vi "Update Values VI.vi"(4 "Project Ref":refnum<vi>, 6 "Names":string[](array[string]), 7 "Entity Paths":T1, 8 "error in (no error)":errorcluster) -> (0 "error":errorcluster)   [LabVIEW 2020, in "Conditum-Tools.lvlib" / "Entity Editor.lvclass"]
uses:
  Entity Editor.lvclass
  Entity Paths.ctl
  <vilib>/Utility/miscctls.llb/LVPositionTypeDef.ctl
  <vilib>/Utility/traverseref.llb/TRef TravTarget.ctl
  <vilib>/IlluminatedG/IG Conditum Base/Conditum/Columns/Type/Copy Value.vi
  <vilib>/Utility/traverseref.llb/VI Scripting - Traverse.lvlib
  <vilib>/IlluminatedG/IG Conditum Base/Conditum/Columns/Type/Type.lvclass
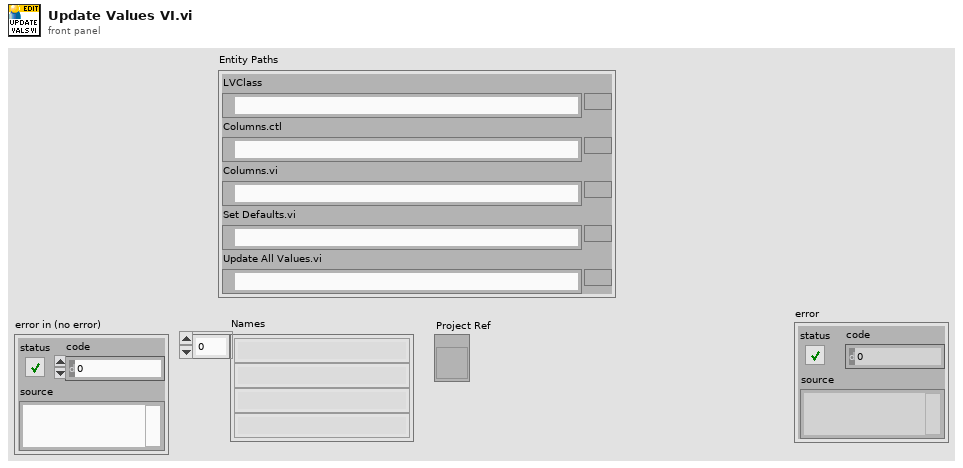
[diagram p1: front panel]
types:
  T1 = typedef "Conditum-Tools.lvlib/Entity Editor.lvclass/Entity Paths.ctl" = cluster{"LVClass":path, "Columns.ctl":path, "Columns.vi":path, "Set Defaults.vi":path, "Update All Values.vi":path}
  T2 = typedef "TRef TravTarget.ctl" = enum16{"FP", "BD", "Other"}
  T3 = typedef "LVPositionTypeDef.ctl" = cluster{"Left":i32, "Top":i32}
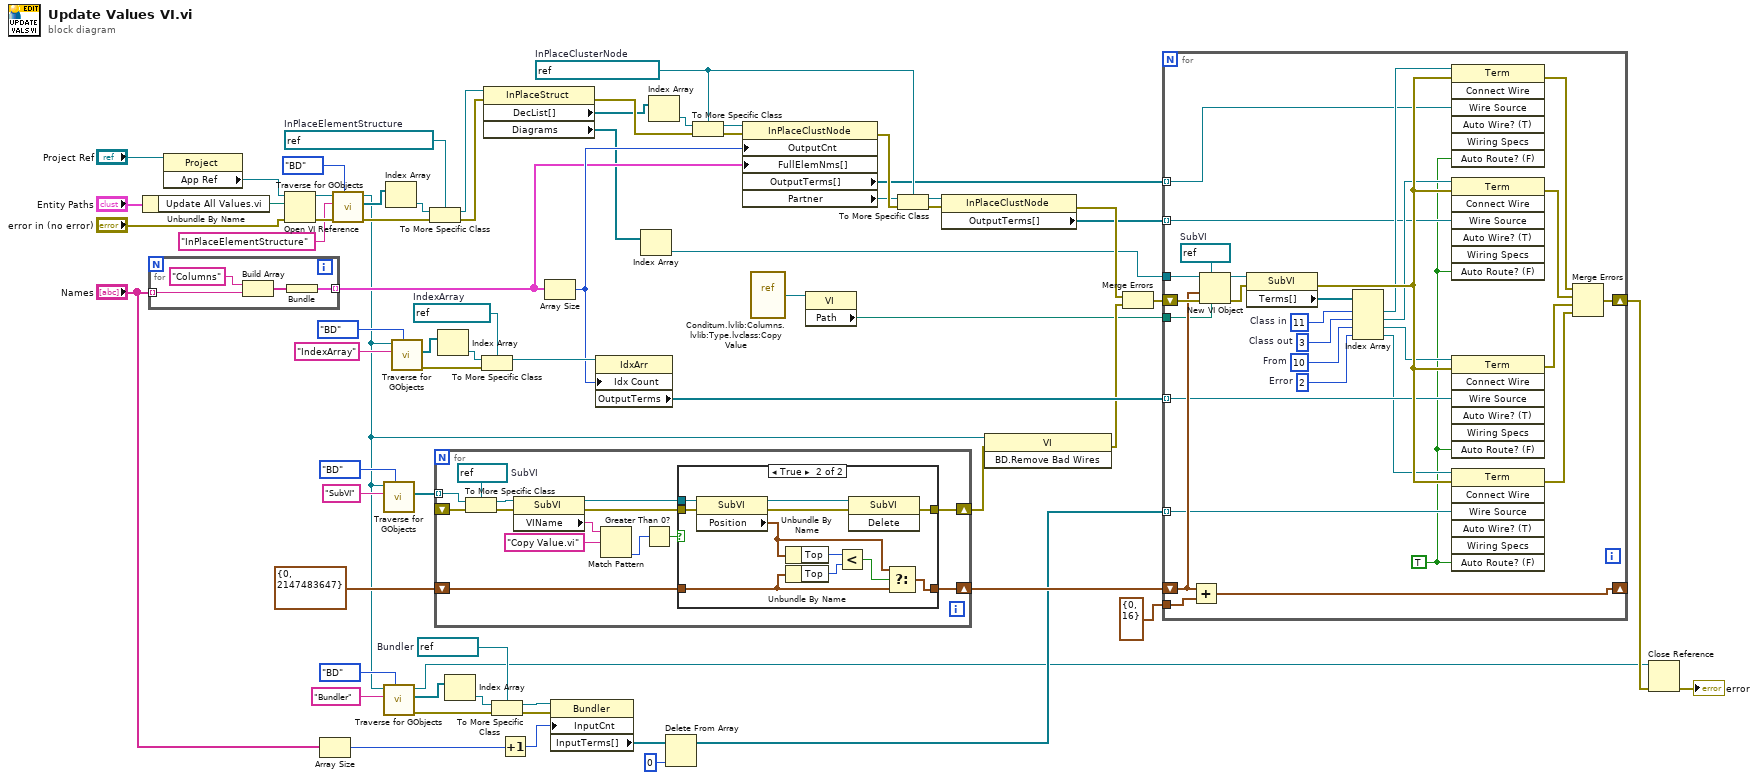
[diagram p0: block diagram]
diagram:
  w15 = refnum<vi> refnum  # Bundler
  w42 = refnum<vi> refnum  # IndexArray
  w36 = refnum<vi> refnum  # InPlaceClusterNode
  w53 = refnum<vi> refnum  # InPlaceElementStructure
  n1 = Unbundle By Name("Entity Paths") -> ("Update All Values.vi"=w62:path)
  n2 = for {
    tunnel: "Names" -> [w73] mode=indexing
    tunnel: [w70] -> w39 mode=indexing
    n3 = Build Array("Columns" ("element"), w73) -> (w71:string[])
    n4 = Bundle(w71) -> (w70:cluster{string[]})  [unwired: 1 in]
  }
  n5 = property class="Project"(reference="Project Ref") -> ("App Ref"=w60:refnum<vi>)  [unwired: 1 in, 2 out]
  n6 = Open VI Reference(application reference (local)=w60, vi path=w62, error in (no error)="error in (no error)") -> (vi reference=w59:refnum<vi>, error out=w58:errorcluster)  [unwired: 3 in]
  n7 = Array Size(array="Names") -> (size(s)=w11:i32)
  n8 = call <vilib>:"Traverse for GObjects.vi"("Traverse Target"=TRef_TravTarget."BD", "error in (no error)"=w58, "Class Name"="InPlaceElementStructure", "VI Refnum"=w59) -> ("error out"=w51:errorcluster, "References"=w55:refnum<vi>[], "dup VI Refnum"=w1:refnum<vi>)  [unwired: 4 in, 1 out]
  n9 = call <vilib>:"Traverse for GObjects.vi"("Traverse Target"=TRef_TravTarget."BD", "Class Name"="SubVI", "VI Refnum"=w1) -> ("References"=w27:refnum<vi>[])  [unwired: 5 in, 3 out]
  n10 = call <vilib>:"Traverse for GObjects.vi"("Traverse Target"=TRef_TravTarget."BD", "Class Name"="Bundler", "VI Refnum"=w1) -> ("error out"=w16:errorcluster, "References"=w18:refnum<vi>[], "dup VI Refnum"=w5:refnum<vi>)  [unwired: 5 in, 1 out]
  n11 = Index Array(array=w55) -> (element=w54:refnum<vi>)  [unwired: 1 in]
  n12 = call <vilib>:"Traverse for GObjects.vi"("Traverse Target"=TRef_TravTarget."BD", "Class Name"="IndexArray", "VI Refnum"=w1) -> ("error out"=w43:errorcluster, "References"=w44:refnum<vi>[])  [unwired: 5 in, 2 out]
  n13 = To More Specific Class(target class=w53, reference=w54, error in=w51) -> (specific class reference=w52:refnum<vi>, error out=w50:errorcluster)
  n14 = for {
    tunnel: w27 -> [w85] mode=indexing
    shift-right: [w87] -> w25
    shift-left: _ -> [w86]
    shift-right: [w74] -> w26
    shift-left: T3 {"Left"=0, "Top"=2147483647} ("Position") -> [w75]
    w84 = refnum<vi> refnum  # SubVI
    n15 = To More Specific Class(target class=w84, reference=w85, error in=w86) -> (specific class reference=w83:refnum<vi>, error out=w82:errorcluster)
    n16 = property class="SubVI"(reference=w83, error in=w82) -> (reference out=w77:refnum<vi>, error out=w76:errorcluster, "VIName"=w81:string)
    n17 = Match Pattern(string=w81, regular expression="Copy Value.vi") -> (offset past match=w79:i32)  [unwired: 1 in, 3 out]
    n18 = Greater Than 0?(x=w79) -> (x > 0?=w78:bool)
    n19 = case shown="True" w78 {
      tunnel: [w89 w100] -> w87
      tunnel: w77 -> [_ w99]
      tunnel: w76 -> [w89 w98]
      tunnel: w75 -> [w88 w93]
      tunnel: [w88 w90] -> w74
      frame False {
      }
      frame True {
        n20 = property class="SubVI"(reference=w99, error in=w98) -> (reference out=w97:refnum<vi>, error out=w96:errorcluster, "Position"=w92:T3)
        n21 = Unbundle By Name(w92) -> ("Top"=w95:i32)
        n22 = Unbundle By Name(w93) -> ("Top"=w94:i32)
        n23 = Less?(x=w95, y=w94) -> (x < y?=w91:bool)
        n24 = invoke class="SubVI" method="Delete"(reference=w97, error in=w96) -> (error out=w100:errorcluster)  [unwired: 1 in, 2 out]
        n25 = Select(t=w92, s=w91, f=w93) -> (s? t:f=w90:T3)
      }
    }
  }
  n26 = Index Array(array=w44) -> (element=w45:refnum<vi>)  [unwired: 1 in]
  n27 = Index Array(array=w18) -> (element=w17:refnum<vi>)  [unwired: 1 in]
  n28 = To More Specific Class(target class=w42, reference=w45, error in=w43) -> (specific class reference=w41:refnum<vi>)  [unwired: 1 out]
  n29 = property class="InPlaceStruct"(reference=w52, error in=w50) -> (error out=w67:errorcluster, "DecList[]"=w66:refnum<vi>[], "Diagrams"=w3:refnum<vi>[])  [unwired: 1 out]
  n30 = To More Specific Class(target class=w15, reference=w17, error in=w16) -> (specific class reference=w14:refnum<vi>, error out=w13:errorcluster)
  n31 = Increment(x=w11) -> (x+1=w10:i32)
  n32 = Array Size(array=w39) -> (size(s)=w40:i32)
  n33 = property class="Bundler"(reference=w14, error in=w13, "InputCnt"=w10) -> ("InputTerms[]"=w9:refnum<vi>[])  [unwired: 2 out]
  n34 = property class="IdxArr"(reference=w41, "Idx Count"=w40) -> ("OutputTerms"=w32:refnum<vi>[])  [unwired: 1 in, 2 out]
  n35 = Index Array(array=w3) -> (element=w2:refnum<vi>)  [unwired: 1 in]
  n36 = Index Array(array=w66) -> (element=w65:refnum<vi>)  [unwired: 1 in]
  n37 = Delete From Array(array=w9, index=0) -> (array with subset deleted=w8:refnum<vi>[])  [unwired: 1 in, 1 out]
  n38 = To More Specific Class(target class=w36, reference=w65, error in=w67) -> (specific class reference=w64:refnum<vi>, error out=w49:errorcluster)
  n39 = property class="InPlaceClustNode"(reference=w64, error in=w49, "OutputCnt"=w40, "FullElemNms[]"=w39) -> (error out=w68:errorcluster, "OutputTerms[]"=w33:refnum<vi>[], "Partner"=w38:refnum<vi>)  [unwired: 1 out]
  n40 = vi-ref "Conditum.lvlib:Columns.lvlib:Type.lvclass:Copy Value.vi"() -> (w31:refnum<vi>)
  n41 = property class="VI"(reference=w31) -> ("Path"=w21:path)  [unwired: 1 in, 2 out]
  n42 = To More Specific Class(target class=w36, reference=w38, error in=w68) -> (specific class reference=w37:refnum<vi>, error out=w35:errorcluster)
  n43 = property class="InPlaceClustNode"(reference=w37, error in=w35) -> (error out=w69:errorcluster, "OutputTerms[]"=w34:refnum<vi>[])  [unwired: 1 out]
  n44 = invoke class="VI" method="BD.Remove Bad Wires"(reference=w1, error in=w25) -> (error out=w22:errorcluster)  [unwired: 1 in, 2 out]
  n45 = Merge Errors(w69, w22) -> (w23:errorcluster)
  n46 = for {
    tunnel: w34 -> [w111] mode=indexing
    tunnel: w33 -> [w113] mode=indexing
    tunnel: w32 -> [w110] mode=indexing
    shift-right: [w126] -> _
    shift-left: w26 -> [w124]
    tunnel: T3 {"Left"=0, "Top"=16} ("Position") -> [w127]
    shift-right: [w103] -> w6
    shift-left: w23 -> [w128]
    tunnel: w2 -> [w125]
    tunnel: w21 -> [w123]
    tunnel: w8 -> [w107] mode=indexing
    w106 = TRUE ("Auto Route? (F)")
    w115 = 2  # Error
    w116 = 10  # From
    w117 = 3  # Class out
    w118 = 11  # Class in
    w122 = refnum<vi> refnum  # SubVI
    n47 = Add(x=w124, y=w127) -> (x+y=w126:T3)
    n48 = New VI Object(vi object class=w122, owner refnum=w125, position/next to=w124, 6:w123, 8:w128) -> (object refnum=w121:refnum<vi>, 0:w120:errorcluster)  [unwired: 3 in]
    n49 = property class="SubVI"(reference=w121, error in=w120) -> (error out=w129:errorcluster, "Terms[]"=w119:refnum<vi>[])  [unwired: 1 out]
    n50 = Index Array(array=w119, index #1=w118, index #2=w117, index #3=w116, index #4=w115) -> (element #1=w114:refnum<vi>, element #2=w112:refnum<vi>, element #3=w109:refnum<vi>, element #4=w108:refnum<vi>)
    n51 = invoke class="Term" method="Connect Wire"(reference=w114, error in=w129, "Wire Source"=w113, "Auto Route? (F)"=w106) -> (error out=w104:errorcluster)  [unwired: 3 in, 6 out]
    n52 = invoke class="Term" method="Connect Wire"(reference=w112, error in=w129, "Wire Source"=w111, "Auto Route? (F)"=w106) -> (error out=w105:errorcluster)  [unwired: 3 in, 6 out]
    n53 = invoke class="Term" method="Connect Wire"(reference=w109, error in=w129, "Wire Source"=w110, "Auto Route? (F)"=w106) -> (error out=w102:errorcluster)  [unwired: 3 in, 6 out]
    n54 = invoke class="Term" method="Connect Wire"(reference=w108, error in=w129, "Wire Source"=w107, "Auto Route? (F)"=w106) -> (error out=w101:errorcluster)  [unwired: 3 in, 6 out]
    n55 = Merge Errors(w104, w105, w102, w101) -> (w103:errorcluster)
  }
  n56 = Close Reference(reference=w5, error in (no error)=w6) -> (error out=→"error":errorcluster)
